vi "Get All Panels.vi"(8 "error in (no error)":errorcluster, 11 "Manager in":refnum<class "Manager.lvclass">) -> (0 "error out":errorcluster, 2 "Panels":refnum<class "Panel.lvclass">[](array[class]), 3 "Manager out":refnum<class "Manager.lvclass">)   [LabVIEW 2020, in "OOPanel.lvlib" / "Manager.lvclass"]
uses:
  Manager.lvclass
  Panel/Panel.lvclass
  Manager.lvclass/Manager.ctl
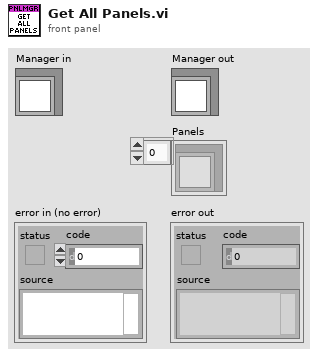
[diagram p1: front panel]
types:
  T1 = typedef "OOPanel.lvlib/Manager.lvclass/Ref Data.ctl" = cluster{"SubPanel Map":T2, "Panels":refnum<class "Panel.lvclass">[]}
  T2 = typedef "OOPanel.lvlib/Manager.lvclass/SubPanel Map.ctl" = cluster{"SubPanels":refnum<vi>[], "Panels":refnum<class "Panel.lvclass">[]}
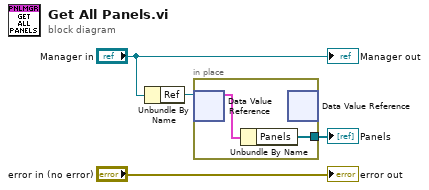
[diagram p0: block diagram]
diagram:
  n1 = Unbundle By Name("Manager in") -> ("Ref"=w3:refnum<data-value>)
  n2 = in-place {
    in-place-border: [w5] -> w1
    n3 = in-place-dvr #1(w3) -> (w6:T1)  [unwired: 1 out]
    n4 = Unbundle By Name(w6) -> ("Panels"=w5:refnum<class "Panel.lvclass">[])
    n5 = in-place-dvr #1() -> ()  [unwired: 1 in, 2 out]
  }
  "Panels" <- w1
  "error out" <- "error in (no error)"
  "Manager out" <- "Manager in"
